vi "veristandSteps-installer-commandLineArgs.vi"(8 "error in (no error)":errorcluster, 10 "New Command Line Argument(s)":string, 11 "InstallerMutationSession":T1={"Installer Build Specification Ref"=refnum, "Project reference out"=refnum, "Installer Project Path"=path "C:/Users/Public/Documents/Git-Source/VeriStand-Custom-Steps-For-TestStand/Source/LabVIEW Code/Installer/Installer - Copy.lvproj"}) -> (0 "error out":errorcluster, 3 "InstallerMutationSession out":T1={"Installer Build Specification Ref"=refnum, "Project reference out"=refnum, "Installer Project Path"=path "C:/Users/Public/Documents/Git-Source/VeriStand-Custom-Steps-For-TestStand/Source/LabVIEW Code/Installer/Installer - Copy.lvproj"})   [LabVIEW 2014, in "veristand-steps-build-system.lvlib"]
uses:
  veristand-steps-build-system.lvlib
  lv-build-system/types/LVInstallerMutationSession.ctl
  lv-build-system/lv-build-library.lvlib
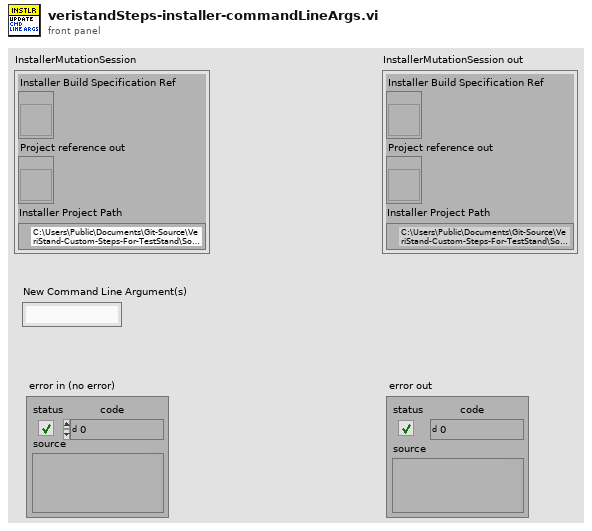
[diagram p1: front panel]
types:
  T1 = typedef "lv-build-library.lvlib/LVInstallerMutationSession.ctl" = cluster{"Installer Build Specification Ref":refnum<vi>, "Project reference out":refnum<vi>, "Installer Project Path":path}
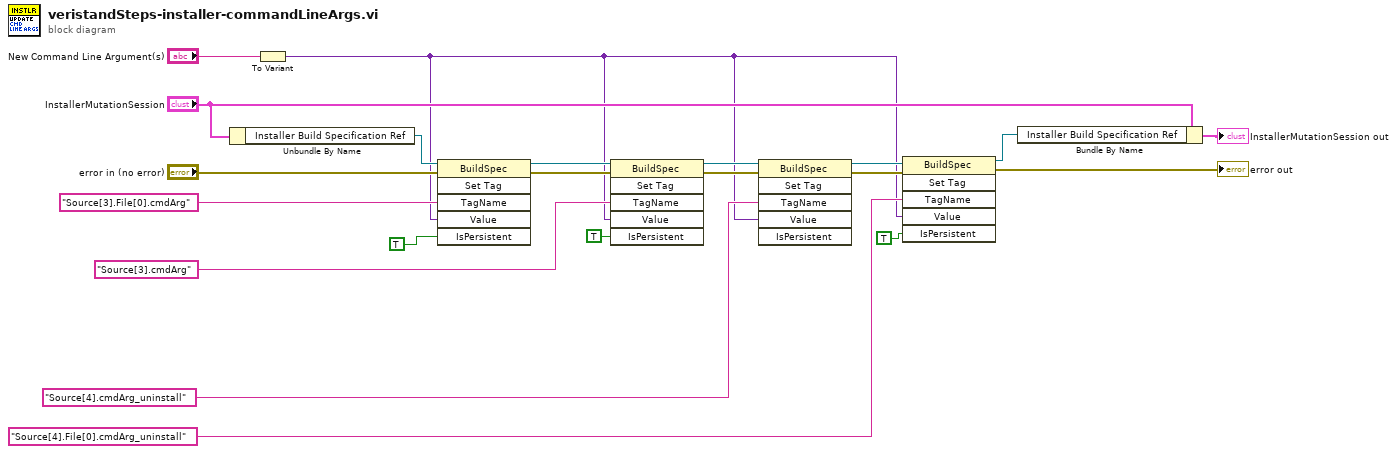
[diagram p0: block diagram]
diagram:
  n1 = Unbundle By Name("InstallerMutationSession") -> ("Installer Build Specification Ref"=w18:refnum<vi>)
  n2 = To Variant(anything="New Command Line Argument(s)") -> (Variant=w1:variant)
  n3 = invoke class="BuildSpec" method="Set Tag"(reference=w18, error in="error in (no error)", "TagName"="Source[3].File[0].cmdArg" ("Tag Name"), "Value"=w1, "IsPersistent"=TRUE ("Is Persistent")) -> (reference out=w10:refnum<vi>, error out=w9:errorcluster)  [unwired: 1 in, 4 out]
  n4 = invoke class="BuildSpec" method="Set Tag"(reference=w10, error in=w9, "TagName"="Source[3].cmdArg" ("Tag Name"), "Value"=w1, "IsPersistent"=TRUE ("Is Persistent")) -> (reference out=w6:refnum<vi>, error out=w5:errorcluster)  [unwired: 1 in, 4 out]
  n5 = invoke class="BuildSpec" method="Set Tag"(reference=w6, error in=w5, "TagName"="Source[4].cmdArg_uninstall" ("Tag Name"), "Value"=w1) -> (reference out=w3:refnum<vi>, error out=w4:errorcluster)  [unwired: 2 in, 4 out]
  n6 = invoke class="BuildSpec" method="Set Tag"(reference=w3, error in=w4, "TagName"="Source[4].File[0].cmdArg_uninstall" ("Tag Name"), "Value"=w1, "IsPersistent"=TRUE ("Is Persistent")) -> (reference out=w13:refnum<vi>, error out=→"error out":errorcluster)  [unwired: 1 in, 4 out]
  n7 = Bundle By Name(cluster="InstallerMutationSession", "Installer Build Specification Ref"=w13) -> (→"InstallerMutationSession out":T1)
